vi "Symphony Set Trigger.vi"(6 "SigType":T1(ring), 7 "Trigger On/Off":bool, 8 "error in (no error)":errorcluster, 9 "Event":T2(ring), 10 "TrigAddress":i32, 11 "JYCCDLib.IJYCCDReqd":refnum<k7>) -> (0 "error out":errorcluster, 3 "JYCCDLib.IJYCCDReqd":refnum<k7>)   [LabVIEW 2012]
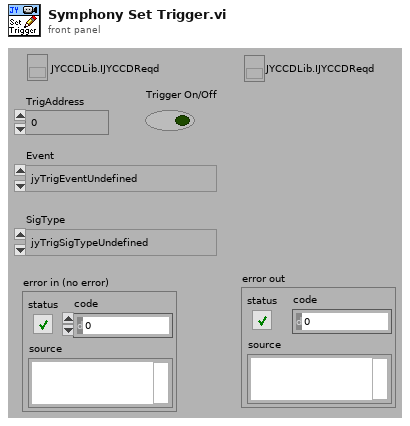
[diagram p1: front panel]
types:
  T1 = enum16{"jyTrigSigTypeUndefined", "jyTrigSigTypeTTLHigh", "jyTrigSigTypeTTLLow"}
  T2 = enum16{"jyTrigEventUndefined", "jyTrigEventOnStart", "jyTrigEventOnEnd", "jyTrigEventPerAccumulation", "jyTrigEventPerCycle", "jyTrigEventPerAcquisition", "jyTrigEventPerRegion", "jyTrigEventScanStart"}
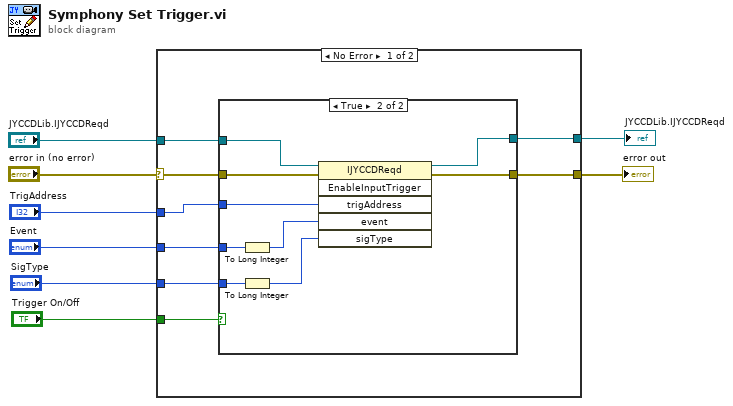
[diagram p0: block diagram]
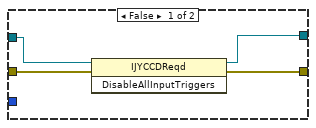
[diagram p2: hidden frame]
diagram:
  n1 = case shown="No Error" "error in (no error)" {
    selector: "error in (no error)" -> [w10 w30]
    tunnel: "JYCCDLib.IJYCCDReqd" -> [w16 w31]
    tunnel: [w15 w30] -> w7
    tunnel: [w14 w31] -> w6
    tunnel: "TrigAddress" -> [w13 _]
    tunnel: "SigType" -> [w12 _]
    tunnel: "Event" -> [w11 _]
    tunnel: "Trigger On/Off" -> [w9 _]
    frame No Error {
      n2 = case shown="True" w9 {
        tunnel: w16 -> [w20 w29]
        tunnel: [w18 w28] -> w15
        tunnel: [w17 w27] -> w14
        tunnel: w13 -> [_ w26]
        tunnel: w12 -> [_ w25]
        tunnel: w11 -> [_ w24]
        tunnel: w10 -> [w19 w23]
        frame False {
          n3 = invoke class="IJYCCDReqd" method="DisableAllInputTriggers"(reference=w20, error in=w19) -> (reference out=w17:refnum<k7>, error out=w18:errorcluster)  [unwired: 1 in, 1 out]
        }
        frame True {
          n4 = To Long Integer(number=w24) -> (32bit integer=w22:i32)
          n5 = To Long Integer(number=w25) -> (32bit integer=w21:i32)
          n6 = invoke class="IJYCCDReqd" method="EnableInputTrigger"(reference=w29, error in=w23, "trigAddress"=w26, "event"=w22, "sigType"=w21) -> (reference out=w27:refnum<k7>, error out=w28:errorcluster)  [unwired: 1 in, 4 out]
        }
      }
    }
    frame Error {
    }
  }
  "JYCCDLib.IJYCCDReqd" <- w6
  "error out" <- w7
